vi "Parse EST Clusters into EST IP.vi"(8 "error in (no error)":errorcluster, 9 "EST version enum":T1, 10 "EPS IP LUT":variant, 11 "Item Ref in":T2 format="%.0x") -> (0 "error out":errorcluster, 2 "APUs":string[](array[string]), 3 "Item Ref out":T2 format="%.0x")   [LabVIEW 2013, in "Engine Simulation Toolkit System Explorer.lvlib"]
uses:
  Engine Simulation Toolkit System Explorer.lvlib
  <vilib>/NI Veristand/Custom Device API/Custom Device Item Ref.ctl
  Shared/Bitfile EST Version.ctl
  Shared/Properties.vi
  <vilib>/NI Veristand/Custom Device API/Set Item Property (String Array).vi
  Shared/Engine Simulation Toolkit Shared.lvlib
  <vilib>/NI Veristand/Custom Device API/Custom Device API.lvlib
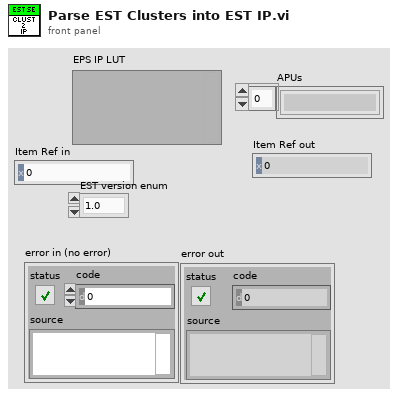
[diagram p1: front panel]
types:
  T1 = typedef "Engine Simulation Toolkit Shared.lvlib/Bitfile EST Version.ctl" = enum16{"1.0", "1.1", "1.2", "1.3"}
  T2 = typedef "Custom Device API.lvlib/Custom Device Item Ref.ctl" = u64
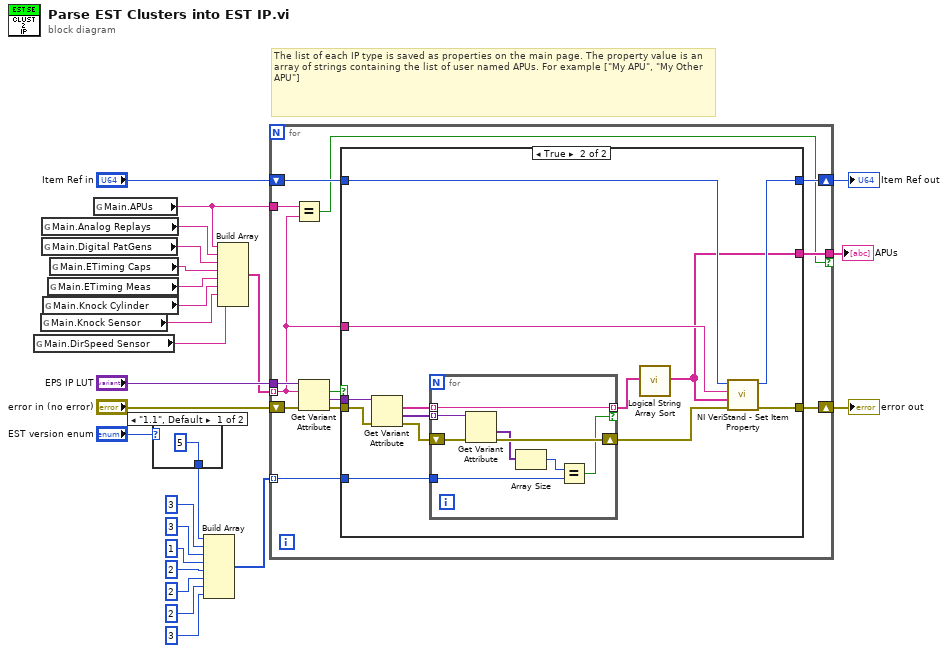
[diagram p0: block diagram]
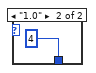
[diagram p2: hidden frame]
diagram:
  # "The list of each IP type is saved as properties on the main page. The property value is an array of strings containing the list of user named APUs. For example [\"My APU\", \"My Other APU\"]"
  n1 = global read "Properties.vi" "Main.DirSpeed Sensor"() -> (w3:string)
  n2 = global read "Properties.vi" "Main.Knock Sensor"() -> (w6:string)
  n3 = global read "Properties.vi" "Main.Analog Replays"() -> (w19:string)
  n4 = global read "Properties.vi" "Main.Digital PatGens"() -> (w18:string)
  n5 = global read "Properties.vi" "Main.Knock Cylinder"() -> (w7:string)
  n6 = global read "Properties.vi" "Main.ETiming Meas"() -> (w16:string)
  n7 = global read "Properties.vi" "Main.ETiming Caps"() -> (w17:string)
  n8 = global read "Properties.vi" "Main.APUs"() -> (w9:string)
  n9 = case shown="\"1.1\", Default" "EST version enum" {
    tunnel: [5 4] -> w20
    frame "1.1", Default {
    }
    frame "1.0" {
    }
  }
  n10 = Build Array(w20, 3, 3, 1, 2, 2, 2, 3) -> (w13:i32[])
  n11 = Build Array(w9, w19, w18, w17, w16, w7, w6, w3) -> (w14:string[])
  n12 = for {
    shift-right: [w35] -> w12
    shift-left: "error in (no error)" -> [w40]
    tunnel: "EPS IP LUT" -> [w39]
    tunnel: w14 -> [w31] mode=indexing
    tunnel: w13 -> [w34] mode=indexing
    shift-right: [w32] -> w10
    shift-left: "Item Ref in" -> [w33]
    tunnel: w9 -> [w30]
    tunnel: [w29] -> w8 if=w28
    n13 = Equal?(x=w30, y=w31) -> (x = y?=w28:bool)
    n14 = Get Variant Attribute(Variant=w39, name=w31, error in=w40) -> (found=w38:bool, value=w36:variant, error out=w37:errorcluster)  [unwired: 1 in, 1 out]
    n15 = case shown="True" w38 {
      tunnel: w37 -> [w41 w54]
      tunnel: w36 -> [_ w55]
      tunnel: [w41 w48] -> w35
      tunnel: w34 -> [_ w53]
      tunnel: w31 -> [_ w47]
      tunnel: w33 -> [w42 w46]
      tunnel: [w42 w45] -> w32
      tunnel: [_ w43] -> w29
      frame False {
      }
      frame True {
        n16 = Get Variant Attribute(Variant=w55, error in=w54) -> (names=w51:string[], values=w50:variant[], error out=w52:errorcluster)  [unwired: 2 in, 1 out]
        n17 = for {
          tunnel: w53 -> [w63]
          shift-right: [w59] -> w49
          shift-left: w52 -> [w60]
          tunnel: w51 -> [w57] mode=indexing
          tunnel: w50 -> [w61] mode=indexing
          tunnel: [w57] -> w44 mode=indexing if=w56
          n18 = Get Variant Attribute(Variant=w61, error in=w60) -> (values=w58:variant[], error out=w59:errorcluster)  [unwired: 2 in, 2 out]
          n19 = Array Size(array=w58) -> (size(s)=w62:i32)
          n20 = Equal?(x=w62, y=w63) -> (x = y?=w56:bool)
        }
        n21 = call "Logical String Array Sort.vi"("Unsorted List"=w44) -> ("Sorted List"=w43:string[])  [unwired: 18 in]
        n22 = call-poly <vilib>:"NI VeriStand - Set Item Property.vi"("error in (no error)"=w49, "Value"=w43, "Property Name"=w47, "Item Ref in"=w46) -> ("error out"=w48:errorcluster, "Item Ref out"=w45:T2)  [unwired: 5 in, 1 out]
      }
    }
  }
  "error out" <- w12
  "Item Ref out" <- w10
  "APUs" <- w8
